vi "Process.vi"(7 "MQTT_Base in":refnum<class "MQTT_Base.lvclass">, 8 "error in (no error)":errorcluster, 10 "Message":refnum<class "PUBLISH.lvclass">, 11 "Server In":refnum<class "MQTT-Server.lvclass">) -> (0 "error out":errorcluster, 2 "Inbound Message":string, 3 "Server Out":refnum<class "MQTT-Server.lvclass">, 5 "MQTT_Base out":refnum<class "MQTT_Base.lvclass">)   [LabVIEW 2023, in "MQTT-Server.lvlib" / "MQTT-Server.lvclass"]
uses:
  MQTT-Server.lvclass
  <vilib>/LabVIEW Open Source Project/MQTT Control Packets/Control Packets/PUBLISH/PUBLISH.lvclass
  C:/Program Files/National Instruments/LabVIEW 2023/vi.lib/LabVIEW Open Source Project/MQTT Control Packets/Control Packets/ControlPacket/ControlPacket.lvclass
  <vilib>/LabVIEW Open Source Project/MQTT Connection/MQTT_Base/Base Class/MQTT_Base.lvclass
  MQTT-Client/MQTT-Client/Message.ctl
  MQTT-Server.lvclass/MQTT-Server.ctl
  <vilib>/Utility/miscctls.llb/LVMapReplaceAction.ctl
  <vilib>/LabVIEW Open Source Project/MQTT Control Packets/Control Packets/ControlPacket/ControlPacket.lvclass
  C:/Program Files/National Instruments/LabVIEW 2023/vi.lib/LabVIEW Open Source Project/MQTT Control Packets/Control Packets/PUBLISH/PUBLISH.lvclass
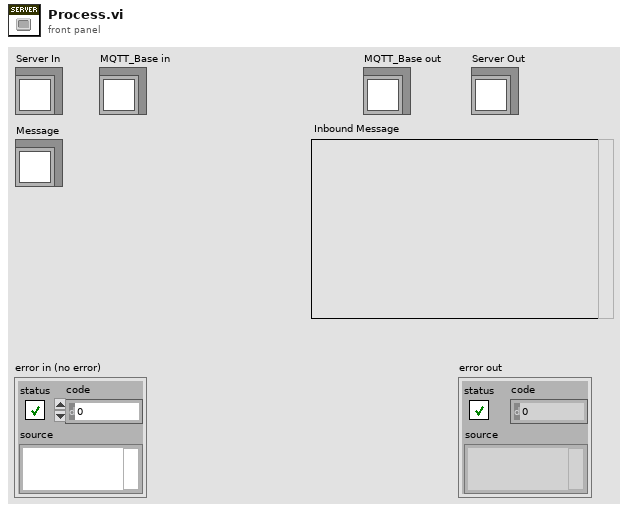
[diagram p1: front panel]
types:
  T1 = typedef "Message.ctl" = cluster{"Time":dbl, "Payload":string}
  T2 = typedef "LVMapReplaceAction.ctl" = enum32{"Modify Entry only if found", "Add or Modify Entry", "Delete Entry"}
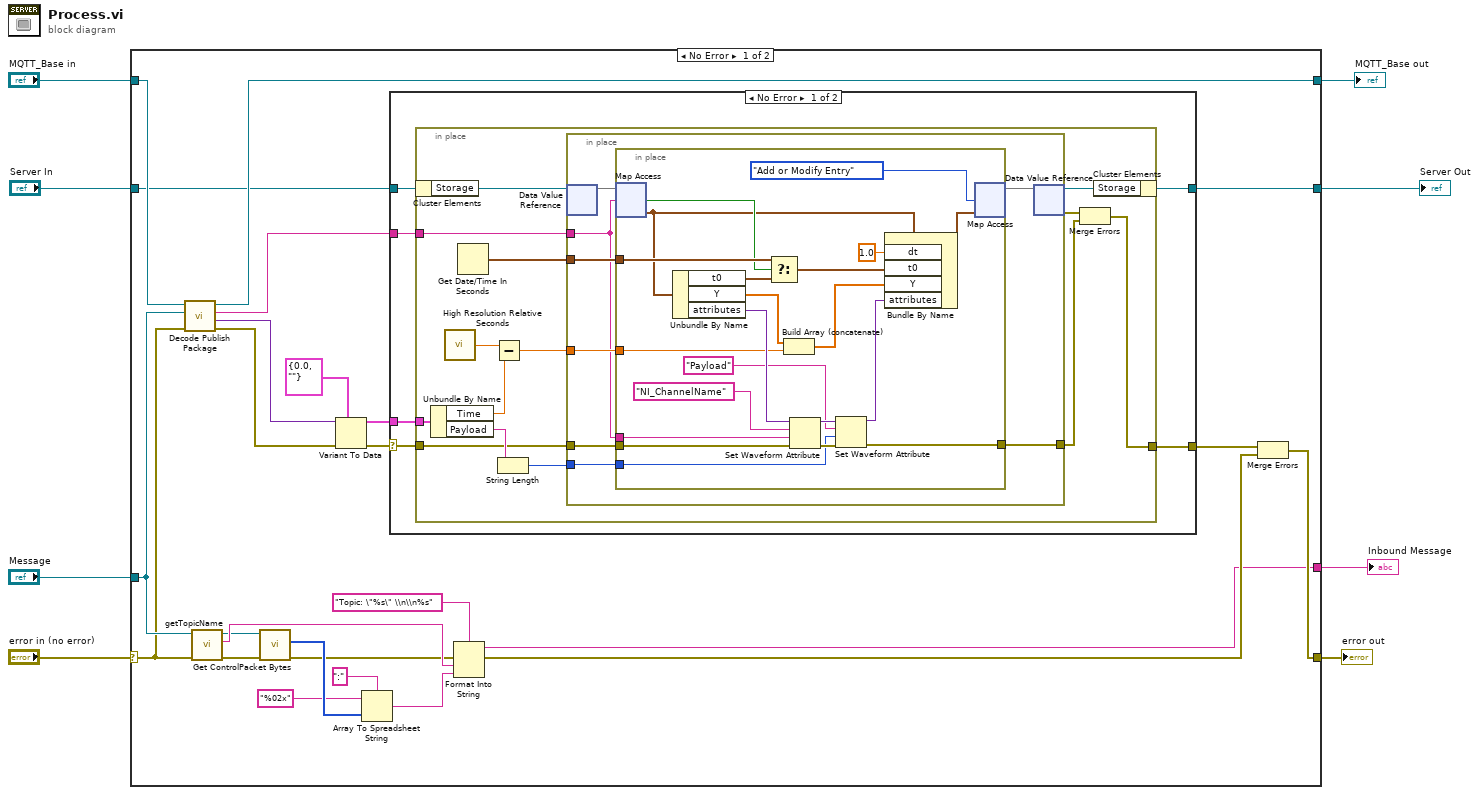
[diagram p0: block diagram]
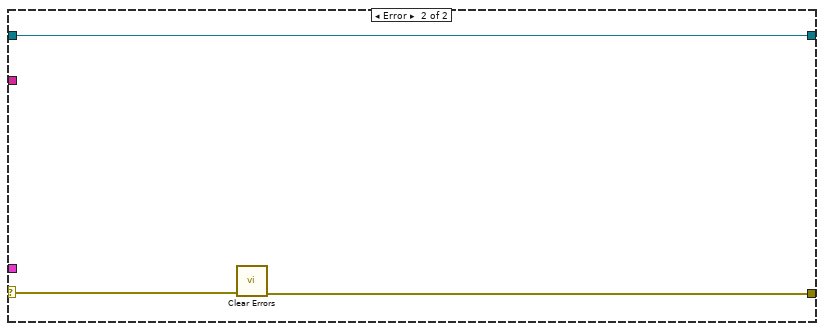
[diagram p2: hidden frame]
diagram:
  n1 = case shown="No Error" "error in (no error)" {
    selector: "error in (no error)" -> [w23 w88]
    tunnel: [w18 w88] -> w7
    tunnel: "MQTT_Base in" -> [w25 w87]
    tunnel: "Message" -> [w24 _]
    tunnel: [w17 w87] -> w4
    tunnel: [w16 _] -> w3
    tunnel: "Server In" -> [w10 w86]
    tunnel: [w9 w86] -> w1
    frame No Error {
      n2 = call <vilib>:"Decode Publish Package.vi"("error in (no error)"=w23, "PUBLISH"=w24, "MQTT_Base in"=w25) -> ("error out"=w27:errorcluster, "Payload"=w26:variant, "Topic"=w11:string, "MQTT_Base out"=w17:refnum<class "MQTT_Base.lvclass">)  [unwired: 5 in]
      n3 = call <vilib>:"getTopicName.vi"("error in (no error)"=w23, "PUBLISH in"=w24) -> ("error out"=w22:errorcluster, "Topic"=w33:string, "PUBLISH out"=w21:refnum<class "PUBLISH.lvclass">)  [unwired: 7 in]
      n4 = call <vilib>:"Get ControlPacket Bytes.vi"("error in (no error)"=w22, "ControlPacket"=w21) -> ("error out"=w20:errorcluster, "Bytes Stream"=w31:u8[])  [unwired: 6 in, 2 out]
      n5 = Variant To Data(error in=w27, type=T1 {"Time"=0.0, "Payload"=""} ("Message"), Variant=w26) -> (data=w13:T1, error out=w14:errorcluster)
      n6 = Array To Spreadsheet String(delimiter (Tab)=":", array=w31, 3:"%02x" ("format string")) -> (spreadsheet string=w28:string)
      n7 = case shown="No Error" w14 {
        selector: w14 -> [w34 w85]
        tunnel: w13 -> [w37 _]
        tunnel: [w35 w84] -> w12
        tunnel: w11 -> [w38 _]
        tunnel: w10 -> [w39 w83]
        tunnel: [w36 w83] -> w9
        frame No Error {
          n8 = in-place {
            in-place-border: w38 -> [w53]
            in-place-border: w37 -> [w52]
            in-place-border: [w40] -> w35
            in-place-border: w34 -> [w43]
            n9 = in-place-cluster #1(w39) -> ("Storage"=w46:refnum<data-value>)
            n10 = Unbundle By Name(w52) -> ("Time"=w50:dbl, "Payload"=w48:string)
            n11 = call <vilib>:"High Resolution Relative Seconds.vi"() -> ("relative seconds"=w51:dbl)
            n12 = Get Date/Time In Seconds() -> (seconds since 1Jan1904=w44:timestamp)
            n13 = Subtract(x=w51, y=w50) -> (x-y=w49:dbl)
            n14 = String Length(string=w48) -> (length=w47:i32)
            n15 = in-place {
              in-place-border: w53 -> [w55]
              in-place-border: w49 -> [w61]
              in-place-border: w47 -> [w60]
              in-place-border: w44 -> [w57]
              in-place-border: w43 -> [w56]
              in-place-border: [w54] -> w41
              n16 = in-place-dvr #2(w46) -> (w59:map{string, waveform(dbl)})  [unwired: 1 out]
              n17 = in-place {
                in-place-border: w61 -> [w72]
                in-place-border: w60 -> [w66]
                in-place-border: w57 -> [w81]
                in-place-border: w56 -> [w73]
                in-place-border: w55 -> [w69]
                in-place-border: [w63] -> w54
                n18 = in-place-map #3(w59, w55) -> (w77:waveform(dbl), w80:bool)  [unwired: 1 in]
                n19 = Unbundle By Name(w77) -> ("t0"=w79:timestamp, "Y"=w71:dbl[], "attributes"=w75:variant)
                n20 = Select(t=w81, s=w80, f=w79) -> (s? t:f=w78:timestamp)
                n21 = Build Array (concatenate)(w71, w72) -> (w70:dbl[])
                n22 = Set Waveform Attribute(4:w73, 5:w69, 6:"NI_ChannelName" ("name"), 7:w75) -> (0:w68:errorcluster, 3:w67:variant)  [unwired: 1 out]
                n23 = Set Waveform Attribute(4:w68, 5:w66, 6:"Payload" ("name"), 7:w67) -> (0:w63:errorcluster, 3:w64:variant)  [unwired: 1 out]
                n24 = Bundle By Name(cluster=w77, "dt"=1.0, "t0"=w78, "Y"=w70, "attributes"=w64) -> (w76:waveform(dbl))
                n25 = in-place-map #3(w76, LVMapReplaceAction."Add or Modify Entry" ("action")) -> (w58:map{string, waveform(dbl)})  [unwired: 2 out]
              }
              n26 = in-place-dvr #2(w58) -> (w45:refnum<data-value>, w42:errorcluster)
            }
            n27 = Merge Errors(w42, w41) -> (w40:errorcluster)
            n28 = in-place-cluster #1("Storage"=w45) -> (w36:refnum<class "MQTT-Server.lvclass">)
          }
        }
        frame Error {
          n29 = call <vilib>:"Clear Errors.vi"("error in (no error)"=w85) -> ("error out"=w84:errorcluster)  [unwired: 5 in, 1 out]
        }
      }
      n30 = Format Into String(format string="Topic: \"%s\" \\n\\n%s", error in=w20, w33, w28) -> (resulting string=w16:string, error out=w19:errorcluster)  [unwired: 1 in]
      n31 = Merge Errors(w12, w19) -> (w18:errorcluster)
    }
    frame Error {
    }
  }
  "error out" <- w7
  "MQTT_Base out" <- w4
  "Inbound Message" <- w3
  "Server Out" <- w1
